vi "Test.vi"() -> ()   [LabVIEW 2019, in "SDL2 Utility.lvlib" / "PS4 Controller.lvclass"]
uses:
  PS4 Controller.lvclass
  LibSDL2 Wrapper/Controls/Joystick Hat Value.ctl
  LibSDL2 Wrapper/Controls/Init Flags.ctl
  PS4 Controller.lvclass/PS4 Controller.ctl
  LibSDL2 Wrapper/LibSDL2.lvlib
panel:
  out "D Pad":T1
  out "Right Stick":cluster{"X":sgl, "Y":sgl, "Button":bool} {"X" scale=-1.0..1.0; "Y" scale=-1.0..1.0}
  out "Left Stick":cluster{"X":sgl, "Y":sgl, "Button":bool} {"X" scale=-1.0..1.0; "Y" scale=-1.0..1.0}
  out "Right Bumper":bool
  out "Left Bumper":bool
  out "Action":T2
  out "Right Trigger":sgl(slide) scale=-1.0..1.0
  out "Left Trigger":sgl(slide) scale=-1.0..1.0
  out "Number Of Joysticks":i32
  out "Loop Period [s]":dbl format="%.1p"
  out "Iteration":i32
  out "Event Type":u32 format="%.0x"
  out "Error":string
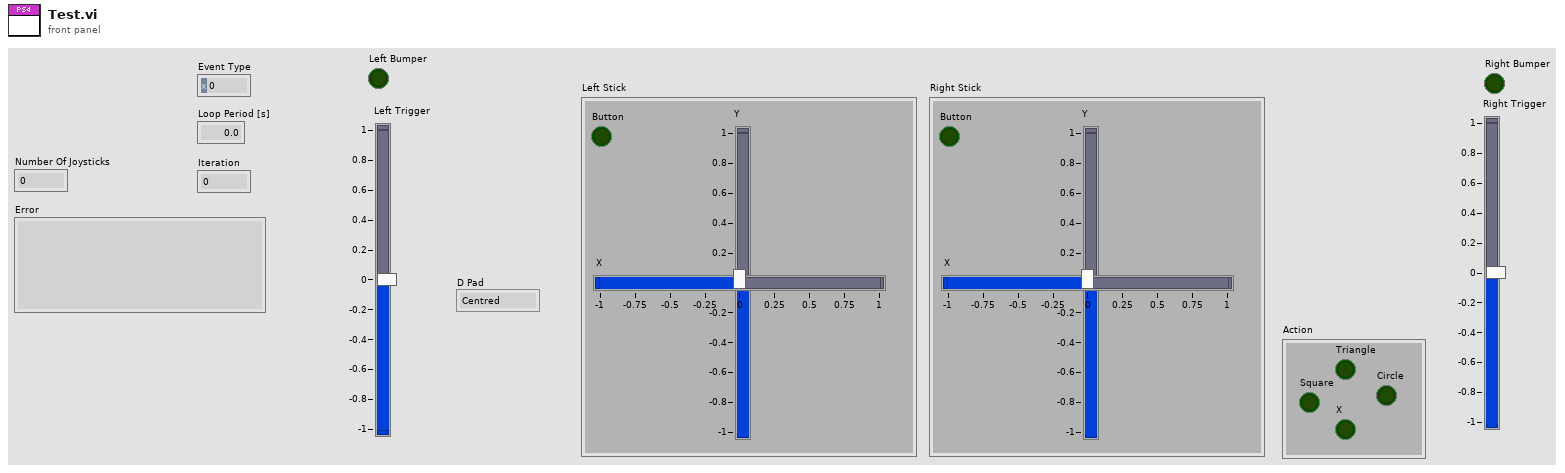
[diagram p1: front panel]
types:
  T1 = typedef "LibSDL2.lvlib/Joystick Hat Value.ctl" = enum16{"Centred", "Up", "Right", "Down", "Left", "Right Up", "Right Down", "Left Up", "Left Down"}
  T2 = cluster{"Triangle":bool, "X":bool, "Square":bool, "Circle":bool}
  T3 = typedef "LibSDL2.lvlib/Init Flags.ctl" = u32
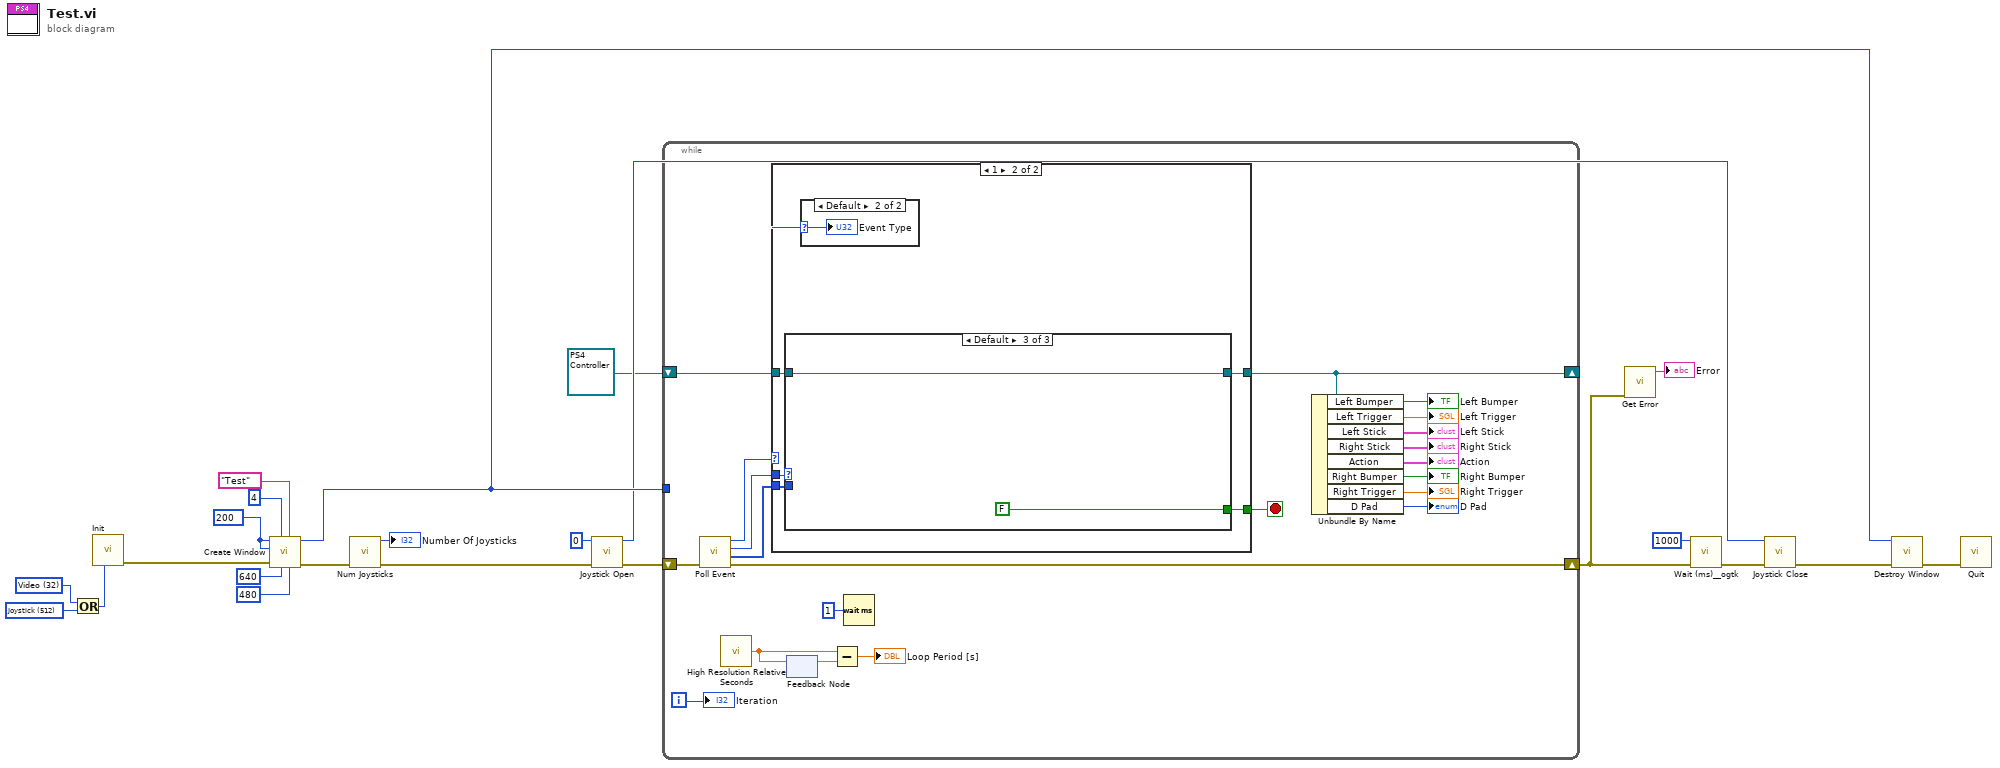
[diagram p0: block diagram]
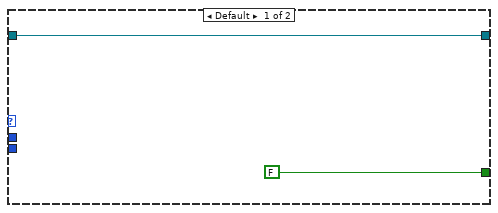
[diagram p2: hidden frame]
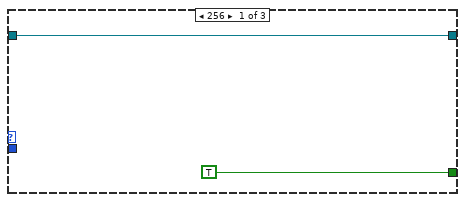
[diagram p4: hidden frame]
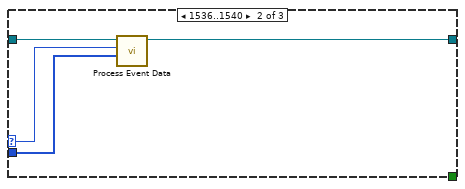
[diagram p5: hidden frame]
diagram:
  w13 = T3 512 items=["Timer"=1, "Audio"=16, "Video"=32, "Joystick"=512, "Haptic"=4096, "Game Controller"=8192, "Events"=16384, "No Parachute"=1048576, "Everything"=17244689] ("Init Flags")
  w10 = T3 32 items=["Timer"=1, "Audio"=16, "Video"=32, "Joystick"=512, "Haptic"=4096, "Game Controller"=8192, "Events"=16384, "No Parachute"=1048576, "Everything"=17244689] ("Init Flags")
  w2 = u32 200 ("Flags")
  n1 = Or(x=w10, y=w13) -> (x .or. y?=w9:T3)
  n2 = call "Init.vi"("Flags"=w9) -> ("error out"=w20:errorcluster)  [unwired: 9 in, 1 out]
  n3 = call "Create Window.vi"("Height"=480, "Title"="Test", "Width"=640, "Flags"=u32 4, "error in"=w20, "Position y"=w2, "Position x"=w2) -> ("error out"=w12:errorcluster, "Window Pointer"=w14:u32)  [unwired: 3 in]
  n4 = call "Num Joysticks.vi"("error in"=w12) -> ("error out"=w8:errorcluster, "Number Of Joysticks"=→"Number Of Joysticks":i32)  [unwired: 9 in]
  n5 = call "Joystick Open.vi"("error in"=w8, "Device Index"=0) -> ("error out"=w7:errorcluster, "Joystick Pointer"=w3:u32)  [unwired: 8 in]
  n6 = while {
    tunnel: w14 -> [_]
    shift-right: [w37] -> w15
    shift-left: w7 -> [w44]
    shift-right: [w32] -> _
    shift-left: refnum<class "PS4 Controller.lvclass"> refnum ("SDL2 Utility.lvlib:PS4 Controller.lvclass") -> [w33]
    i -> [w36]
    stop <- w42 stop-if-true
    n7 = call "Poll Event.vi"("error in"=w44) -> ("error out"=w37:errorcluster, "Event Data"=w43:u8[], "Event Type"=w41:u32, "Return"=w35:i32)  [unwired: 7 in]
    n8 = call <vilib>:"High Resolution Relative Seconds.vi"() -> ("relative seconds"=w40:dbl)
    n9 = case shown="1" w35 {
      tunnel: w43 -> [_ w51]
      tunnel: [FALSE w50] -> w42
      tunnel: w41 -> [_ w49]
      tunnel: w33 -> [w45 w48]
      tunnel: [w45 w47] -> w32
      frame Default {
      }
      frame 1 {
        n10 = case shown="Default" w49 {
          selector: w49 -> [_ w57 _]
          tunnel: w51 -> [_ w56 _]
          tunnel: [TRUE _ FALSE] -> w50
          tunnel: w48 -> [w53 w58 w59]
          tunnel: [w53 w55 w59] -> w47
          frame 256 {
          }
          frame 1536..1540 {
            n11 = call "Process Event Data.vi"("Event Data"=w56, "Event Type"=w57, "PS4 Controller in"=w58) -> ("PS4 Controller out"=w55:refnum<class "PS4 Controller.lvclass">)  [unwired: 8 in]
          }
          frame Default {
          }
        }
        n12 = case shown="Default" w49 {
          selector: w49 -> [_ w52]
          frame 0 {
          }
          frame Default {
            "Event Type" <- w52
          }
        }
      }
    }
    n13 = feedback-in #1(w40) -> ()
    n14 = feedback #1() -> (w39:dbl)  [unwired: 1 in]
    n15 = Subtract(x=w40, y=w39) -> (x-y=→"Loop Period [s]":dbl)
    n16 = Wait (ms)(milliseconds to wait=u32 1) -> ()  [unwired: 1 out]
    n17 = Unbundle By Name(w32) -> ("Left Bumper"=→"Left Bumper":bool, "Left Trigger"=→"Left Trigger":sgl, "Left Stick"=→"Left Stick":cluster{"X":sgl, "Y":sgl, "Button":bool}, "Right Stick"=→"Right Stick":cluster{"X":sgl, "Y":sgl, "Button":bool}, "Action"=→"Action":T2, "Right Bumper"=→"Right Bumper":bool, "Right Trigger"=→"Right Trigger":sgl, "D Pad"=→"D Pad":T1)
    "Iteration" <- w36
  }
  n18 = call "Get Error.vi"("error in"=w15) -> ("Error"=→"Error":string)  [unwired: 9 in, 1 out]
  n19 = call <userlib>:"Wait (ms)__ogtk.vi"("error in (no error)"=w15, "milliseconds to wait"=u32 1000) -> ("error out"=w5:errorcluster)  [unwired: 8 in, 1 out]
  n20 = call "Joystick Close.vi"("error in"=w5, "Joystick Pointer"=w3) -> ("error out"=w4:errorcluster)  [unwired: 9 in]
  n21 = call "Destroy Window.vi"("error in"=w4, "Window Pointer"=w14) -> ("error out"=w17:errorcluster)  [unwired: 9 in]
  n22 = call "Quit.vi"("error in"=w17) -> ()  [unwired: 10 in, 1 out]
